vi "RHA_dialog.vi"(10 "DocFolder":path) -> ()   [LabVIEW 2013, in "RHA.lvlib"]
doc: "<B>Rich Help/About (RHA)</B> provides a tabbed dialog box for displaying information about your LabVIEW application. At a minimum, your application's name and version information should be displayed on the \"About\" tab, but much more information (or links to it) can also be displayed; such as help documentation, version history, EULA, copyright, licensing, plugin information; or any information that you want it to display. It can render plain text files, rich text, markdown files, HTML files, PDF documents, or even image files such as logos."
uses:
  RHA.lvlib
  <userlib>/_OpenG.lib/file/file.llb/Build Path - Traditional__ogtk.vi
  <vilib>/Utility/xml.llb/Read From XML File(string).vi
panel:
  in  "SHDocVw.IWebBrowser2":refnum<k7>(container)
  in  "MainTab":enum32{"About", "Help", "Legal Stuff"}(tab)
  in  "subAbout":T1(tab)
  in  "subHelp":T2(tab)
  in  "subLegalStuff":T3(tab)
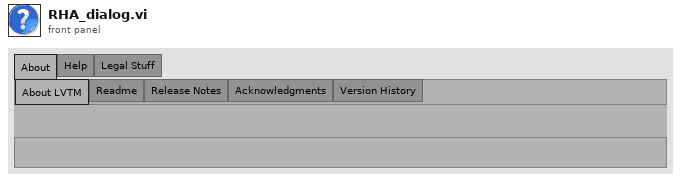
[diagram p1: front panel]
types:
  T1 = enum32{"About LVTM", "Readme", "Release Notes", "Acknowledgments", "Version History"}
  T2 = enum32{"Quick Reference", "Tutorials", "Support"}
  T3 = enum32{"LVTM License (EULA)", "3rd-party Licenses"}
  T4 = cluster{"Control Index":i32, "Control Index":i32}
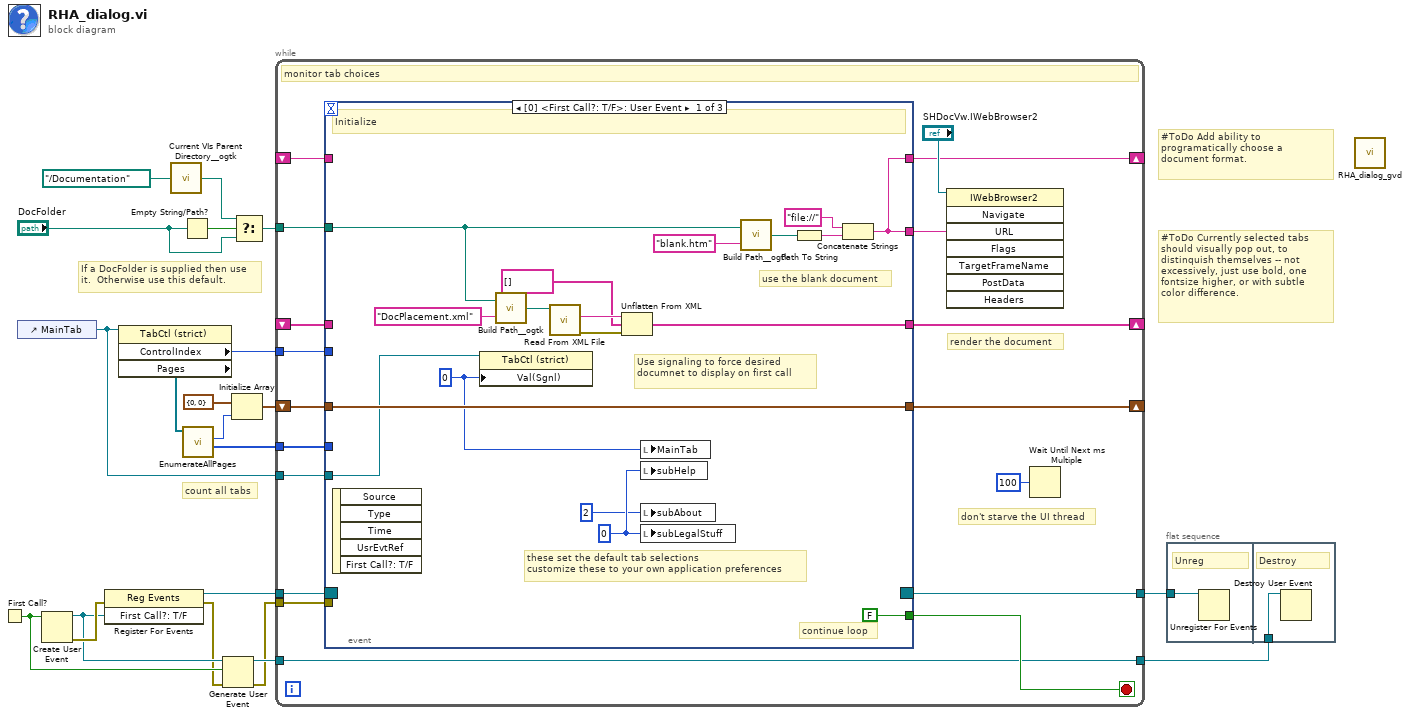
[diagram p0: block diagram]
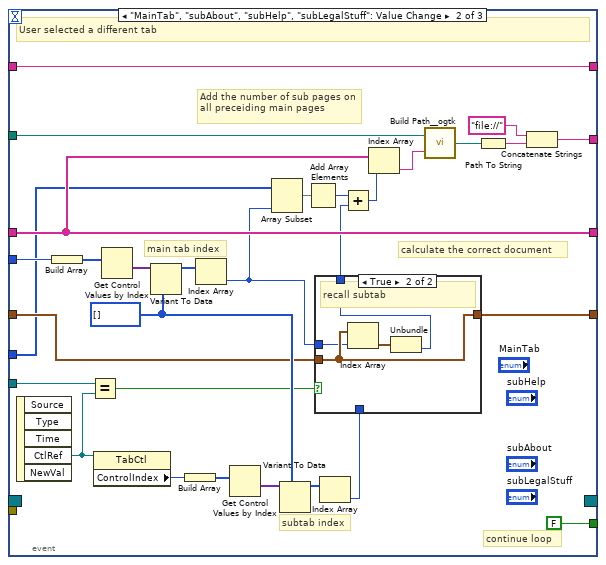
[diagram p2: hidden frame]
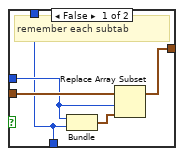
[diagram p3: hidden frame]
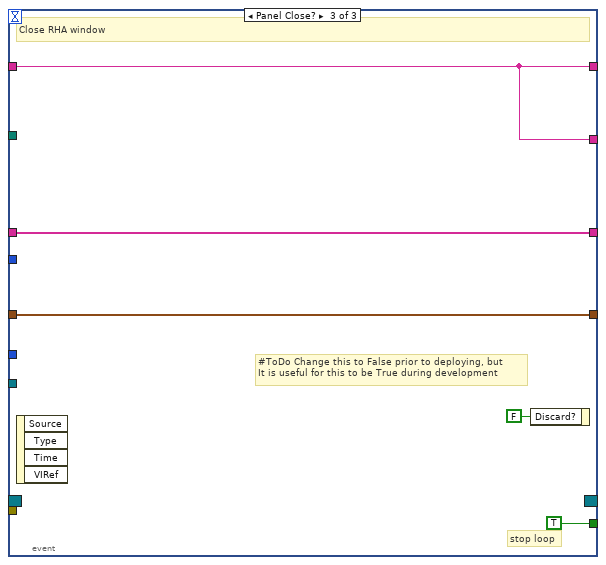
[diagram p4: hidden frame]
diagram:
  # "If a DocFolder is supplied then use it.  Otherwise use this default."
  # "#ToDo Currently selected tabs should visually pop out, to distinquish themselves -- not excessively, just use bold, one fontsize higher, or with subtle color difference."
  # "#ToDo Add ability to programatically choose a document format."
  # "count all tabs"
  n1 = First Call?() -> (First Call?: T/F=w12:bool)
  n2 = control-ref of="MainTab"() -> (w7:refnum<vi>)
  n3 = Create User Event(user event datatype=w12) -> (user event=w14:refnum<user-event>, error out=w15:errorcluster)  [unwired: 1 in]
  n4 = register-events(error in=w15, w14) -> (reference out=w17:refnum<event-registration>, error out=w11:errorcluster)  [unwired: 1 in]
  n5 = property class="TabCtl (strict)"(reference=w7) -> ("ControlIndex"=w8:i32, "Pages"=w6:refnum<vi>[])  [unwired: 1 in, 2 out]
  n6 = call <userlib>:"Current VIs Parent Directory__ogtk.vi"("Relative path (.)"=path "../Documentation" ("name or relative path")) -> ("Parent Directory (+ Relative)"=w19:path)  [unwired: 4 in]
  n7 = Empty String/Path?(string/path="DocFolder") -> (empty?=w21:bool)
  n8 = call "EnumerateAllPages.vi"("Pages"=w6) -> ("#ofSubPages"=w5:i32[], "#ofMainPages"=w4:i32)  [unwired: 6 in, 3 out]
  n9 = Generate User Event(user event=w14, event data cluster=w12, error in=w11) -> (user event out=w13:refnum<user-event>, error out=w10:errorcluster)  [unwired: 1 in]
  n10 = Initialize Array(cluster{"MainIndex":i32, "SubIndex":i32} {"MainIndex"=0, "SubIndex"=0} ("PersistSubtabs"), w4) -> (w3:cluster{"MainIndex":i32, "SubIndex":i32}[])
  n11 = Select(t=w19, s=w21, f="DocFolder") -> (s? t:f=w18:path)
  n12 = while {
    tunnel: w18 -> [w39]
    tunnel: w17 -> [w38]
    tunnel: w10 -> [w37]
    tunnel: [w36] -> w16
    tunnel: w13 -> [w32]
    shift-right: [w34] -> _
    shift-left: _ -> [w33]
    tunnel: [w32] -> w9
    tunnel: w8 -> [w30]
    tunnel: w7 -> [w29]
    tunnel: w5 -> [w28]
    shift-right: [w26] -> _
    shift-left: w3 -> [w27]
    shift-right: [w23] -> _
    shift-left: _ -> [w24]
    stop <- w35 stop-if-true
    # "render the document"
    # "don't starve the UI thread"
    # "monitor tab choices"
    n13 = event shown="[0] <First Call?: T/F>: User Event" {
      selector: w38 -> [_ _ _]
      dyn-events: [_ _ _] -> w36
      timeout: _ -> [_ _ _]
      tunnel: w39 -> [w40 w83 _]
      tunnel: w37 -> [_ _ _]
      tunnel: [w43 w82 w97] -> w22
      tunnel: [FALSE FALSE TRUE] -> w35
      tunnel: [w47 w81 w99] -> w34
      tunnel: w33 -> [_ w81 w99]
      tunnel: w30 -> [_ w68 _]
      tunnel: w29 -> [w42 w72 _]
      tunnel: w28 -> [_ w63 _]
      tunnel: w27 -> [w44 w70 w98]
      tunnel: [w44 w67 w98] -> w26
      tunnel: [w43 w58 w97] -> w23
      tunnel: w24 -> [_ w58 w97]
      event User Event {
        w41 = u32 0
        w46 = u32 0
        # "Use signaling to force desired documnet to display on first call"
        # "use the blank document"
        # "these set the default tab selections\ncustomize these to your own application preferences"
        # "continue loop"
        # "Initialize"
        n14 = event-data() -> ()  [unwired: 1 in, 5 out]
        n15 = property class="TabCtl (strict)"(reference=w42, "Val(Sgnl)"=w41) -> ()  [unwired: 1 in, 2 out]
        n16 = call-poly <userlib>:"Build Path__ogtk.vi"("name or relative path"="DocPlacement.xml" ("XML File Path"), "base path"=w40) -> ("appended path"=w52:path)
        n17 = call-poly <vilib>:"Read From XML File.vi"("XML File Path"=w52) -> ("error out"=w51:errorcluster, "XML Elements"=w50:string)  [unwired: 8 in, 1 out]
        n18 = Unflatten From XML(xml string=w50, type=string[] [], error in (no error)=w51) -> (value=w47:string[])  [unwired: 1 out]
        n19 = local write "MainTab"(w41) -> ()
        n20 = local write "subHelp"(w46) -> ()
        n21 = local write "subAbout"(u32 2) -> ()
        n22 = local write "subLegalStuff"(w46) -> ()
        n23 = call-poly <userlib>:"Build Path__ogtk.vi"("name or relative path"="blank.htm", "base path"=w40) -> ("appended path"=w55:path)
        n24 = Path To String(path=w55) -> (string=w54:string)
        n25 = Concatenate Strings("file://", w54) -> (w43:string)
      }
      event "MainTab", "subAbout", "subHelp", "subLegalStuff": Value Change {
        w71 = i32[] []
        # "calculate the correct document"
        # "Add the number of sub pages on all preceiding main pages"
        # "subtab index"
        # "main tab index"
        # "continue loop"
        # "User selected a different tab"
        n26 = event-data() -> ("CtlRef"=w73:refnum<vi>)  [unwired: 1 in, 4 out]
        n27 = Build Array(w68) -> (w75:i32[])
        n28 = Equal?(x=w72, y=w73) -> (x = y?=w65:bool)
        n29 = property class="TabCtl"(reference=w73) -> ("ControlIndex"=w69:i32)  [unwired: 1 in, 2 out]
        n30 = Get Control Values by Index(1:w75) -> (10:w76:variant[])  [unwired: 2 in, 1 out]
        n31 = Variant To Data(type=w71, Variant=w76) -> (data=w74:i32[])  [unwired: 1 in, 1 out]
        n32 = Build Array(w69) -> (w79:i32[])
        n33 = Index Array(array=w74) -> (element=w62:i32)  [unwired: 1 in]
        n34 = Get Control Values by Index(1:w79) -> (10:w78:variant[])  [unwired: 2 in, 1 out]
        n35 = Array Subset(array=w63, length=w62) -> (w61:i32[])  [unwired: 1 in]
        n36 = Variant To Data(type=w71, Variant=w78) -> (data=w77:i32[])  [unwired: 1 in, 1 out]
        n37 = Add Array Elements(numeric array=w61) -> (sum=w59:i32)
        n38 = Index Array(array=w77) -> (element=w66:i32)  [unwired: 1 in]
        n39 = case shown="True" w65 {
          tunnel: w70 -> [w92 w96]
          tunnel: [w90 w96] -> w67
          tunnel: w62 -> [w89 w95]
          tunnel: w66 -> [w88 _]
          tunnel: [w88 w93] -> w64
          frame False {
            # "remember each subtab"
            n40 = Bundle("Control Index"=w89, "Control Index"=w88) -> (w91:T4)  [unwired: 1 in]
            n41 = Replace Array Subset(array=w92, new element=w91, index=w89) -> (w90:cluster{"MainIndex":i32, "SubIndex":i32}[])
          }
          frame True {
            # "recall subtab"
            n42 = Index Array(array=w96, index=w95) -> (element=w94:cluster{"MainIndex":i32, "SubIndex":i32})
            n43 = Unbundle(w94) -> ("SubIndex"=w93:i32)  [unwired: 1 out]
          }
        }
        n44 = Add(x=w59, y=w64) -> (x+y=w60:i32)
        n45 = Index Array(array=w81, index=w60) -> (element=w80:string)
        n46 = call-poly <userlib>:"Build Path__ogtk.vi"("name or relative path"=w80, "base path"=w83) -> ("appended path"=w85:path)
        n47 = Path To String(path=w85) -> (string=w84:string)
        n48 = Concatenate Strings("file://", w84) -> (w82:string)
      }
      event Panel Close? {
        # "#ToDo Change this to False prior to deploying, but\nIt is useful for this to be True during development"
        # "stop loop"
        # "Close RHA window"
        n49 = event-data() -> ()  [unwired: 1 in, 4 out]
        n50 = event-data("Discard?"=FALSE) -> ()  [unwired: 1 in, 1 out]
      }
    }
    n51 = invoke class="IWebBrowser2" method="Navigate"(reference="SHDocVw.IWebBrowser2", "URL"=w22) -> ()  [unwired: 6 in, 8 out]
    n52 = Wait Until Next ms Multiple(millisecond multiple=u32 100) -> ()  [unwired: 1 out]
  }
  n53 = flat-sequence {
    tunnel: w16 -> [w102]
    tunnel: w9 -> [w103]
    frame #0 {
      # "Unreg"
      n54 = Unregister For Events(event registration refnum=w102) -> ()  [unwired: 1 in, 1 out]
    }
    frame #1 {
      # "Destroy"
      n55 = Destroy User Event(user event=w103) -> ()  [unwired: 1 in, 1 out]
    }
  }
  n56 = call "RHA_dialog_gvd.vi"() -> ()  [unwired: 12 in]
